vi "Pockels Cal-Dialogue on zero entry.vi"(8 "error in (no error)":errorcluster) -> (0 "error out":errorcluster, 1 "Cancelled (Left button pressed)":bool)   [LabVIEW 2020]
doc: "Use this template to create a dialog box with event handling."
uses:
  <vilib>/Utility/miscctls.llb/LVPointTypeDef.ctl
panel:
  in  "Cancel":bool
  in  "Continue":bool
  out "Message":string
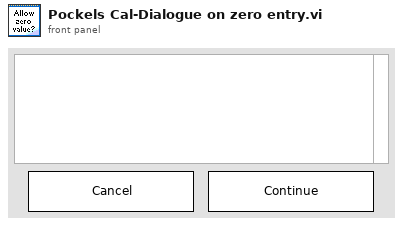
[diagram p1: front panel]
types:
  T1 = typedef "LVPointTypeDef.ctl" = cluster{"Horizontal":i16, "Vertical":i16}
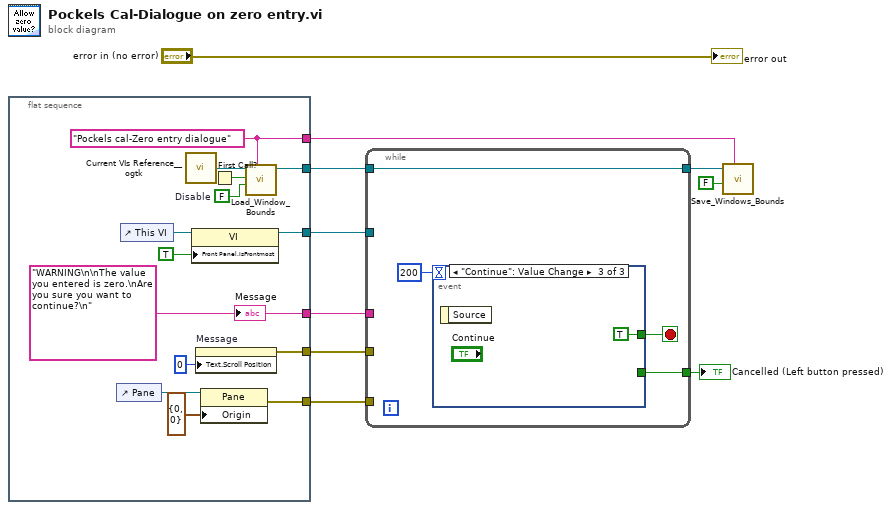
[diagram p0: block diagram]
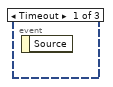
[diagram p2: hidden frame]
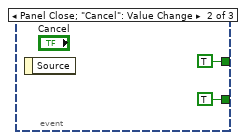
[diagram p3: hidden frame]
diagram:
  n1 = flat-sequence {
    tunnel: [w24] -> w10
    tunnel: [w22] -> w9
    tunnel: [w19] -> w8
    tunnel: [w17] -> w7
    tunnel: [w12] -> w5
    tunnel: [w11] -> w3
    frame #0 {
      w24 = "WARNING\n\nThe value you entered is zero.\nAre you sure you want to continue?\n" ("Message string")
      w13 = FALSE  # Disable
      w12 = "Pockels cal-Zero entry dialogue" ("Window Name (i.e. Key)")
      n2 = control-ref of="Pane"() -> (w16:refnum<vi>)
      n3 = control-ref of="This VI"() -> (w20:refnum<vi>)
      n4 = call <userlib>:"Current VIs Reference__ogtk.vi"() -> ("Current VI's reference"=w15:refnum<vi>)  [unwired: 5 in]
      n5 = property on="Property Node" class="VI"(reference=w20, "Front Panel.IsFrontmost"=TRUE ("Front Panel Window:Is Frontmost")) -> (reference out=w19:refnum<vi>)  [unwired: 1 in, 1 out]
      n6 = property on="Message" class="Str"("Text.Scroll Position"=u32 0) -> (error out=w22:errorcluster)  [unwired: 2 in, 1 out]
      n7 = property class="Pane"(reference=w16, "Origin"=T1 {"Horizontal"=0, "Vertical"=0}) -> (error out=w17:errorcluster)  [unwired: 1 in, 1 out]
      n8 = First Call?() -> (First Call?: T/F=w14:bool)
      n9 = call "Load_Window_Bounds.vi"("Window Name (i.e. Key)"=w12, "Disable"=w13, "First Call"=w14, "Window VI's Ref"=w15) -> ("reference out"=w11:refnum<vi>)  [unwired: 4 in, 3 out]
      "Message" <- w24
    }
  }
  n10 = while {
    tunnel: w10 -> [_]
    tunnel: w9 -> [_]
    tunnel: w7 -> [_]
    tunnel: w8 -> [_]
    tunnel: [w26] -> w6
    tunnel: w3 -> [w25]
    tunnel: [w25] -> w2
    stop <- w28 stop-if-true
    n11 = event shown="[2] \"Continue\": Value Change" {
      selector: _ -> [_ _ _]
      dyn-events: _ -> [_ _ _]
      timeout: 200 -> [_ _ _]
      tunnel: [_ TRUE ("Stop?") TRUE ("Stop?")] -> w28
      tunnel: [_ TRUE ("Stop subpanel") _] -> w26
      event Timeout {
        n12 = event-data() -> ()  [unwired: 1 in, 1 out]
      }
      event Panel Close; "Cancel": Value Change {
        n13 = event-data() -> ()  [unwired: 1 in, 1 out]
      }
      event "Continue": Value Change {
        n14 = event-data() -> ()  [unwired: 1 in, 1 out]
      }
    }
  }
  "Cancelled (Left button pressed)" <- w6
  n15 = call "Save_Windows_Bounds.vi"("Window Name (i.e. Key)"=w5, "Front Panel Window:Open"=FALSE, "Window VI's Ref"=w2) -> ()  [unwired: 8 in, 1 out]
  "error out" <- "error in (no error)"
